vi "Set Read Write T-out.vi"(5 "Write Timeout(in ms)":i32, 7 "Read Timeout(in ms)":i32, 8 "Error In":errorcluster, 11 "SSL Stream":refnum<k24>) -> (0 "Error Out":errorcluster)   [LabVIEW 2014, in "SSL Lib.lvlib"]
doc: "VI Function: This VI sets the time-out for SSL Read and Write operations.\n\nVI Version: 1.0\n\nVI Author: Runjhun Agarwal"
uses:
  <userlib>/SSL Library/SSL Lib.lvlib
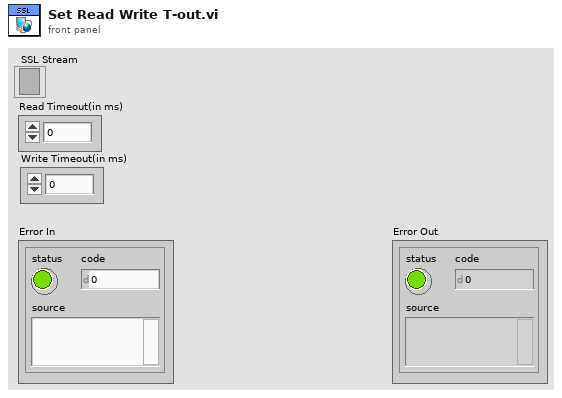
[diagram p1: front panel]
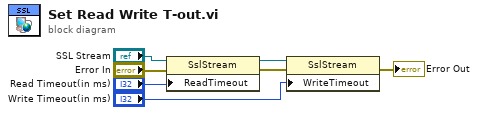
[diagram p0: block diagram]
diagram:
  n1 = property class="SslStream"(reference="SSL Stream", error in="Error In", "ReadTimeout"="Read Timeout(in ms)") -> (reference out=w7:refnum<k24>, error out=w6:errorcluster)
  n2 = property class="SslStream"(reference=w7, error in=w6, "WriteTimeout"="Write Timeout(in ms)") -> (error out=→"Error Out":errorcluster)  [unwired: 1 out]
